vi "ClsGlobalSignalIDmakerforCHRocodileII.vi"(1 "Global Signal Name":i32(ring) items=["StartTime"=64, "Start_PositionX"=65, "Start_PositionY"=66, "Start_PositionZ"=67, "Start_PositionU"=68, "Start_PositionV"=69, "Stop_PositionX"=70, "Stop_PositionY"=71, "Stop_PositionZ"=72, "Stop_PositionU"=73, "Stop_PositionV"=74, "ExposureCount"=75, "ExposureFlags"=76, "RealExpTimeNs"=77, " RealLightingTimeNs"=78, "TriggerLostCounter"=79, "NumberOfValidPeaks"=80, "TicketNumber"=81, "InterferomIntensity"=82, "SampleCounter"=83, " InterfEnergy"=85, " Health_DSPLoad"=86, "Health_Ticketwrongorder"=87, "Health_UPPLostCount"=88, "Health_ExposureLostCount"=89, "Health_UppNotFinished"=90, "PacketTimestampOffset"=91]) -> (0 "Global Signal ID":i32)   [LabVIEW 2015]
doc: "Global Signals ID maker(CHRocodile 2 signal/multichannel devices):\n\nGenerate Signal ID from the Signal Name for Global signals:\n\nGlobal Signal Name[Input]: the global signal name enum input. Global signals appear only once for multichannel/single channel devices for all channels each sample(for example, one sample in a 192-channel device contain only one certain global signal such as the sample counter signal).\n\nGlobal Signal ID[Output]: the calculated global signal ID."
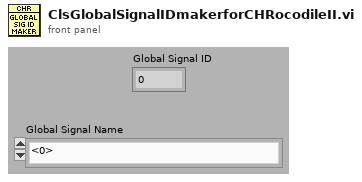
[diagram p1: front panel]
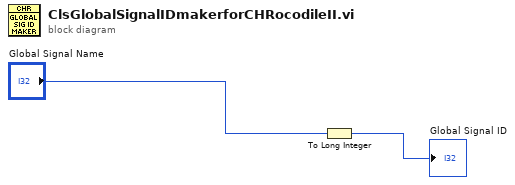
[diagram p0: block diagram]
diagram:
  n1 = To Long Integer(number="Global Signal Name") -> (32bit integer=→"Global Signal ID":i32)
